vi "ep_Build Waveforms (Multiple Lines).vi"(5 "reset? (F)":bool, 6 "current channels":T1[](array[typedef]) {"physical channels"."channel phase" items=["Phase A (L1)", "Phase B (L2)", "Phase C (L3)", "Phase N (Neutral)"]}, 7 "t0":timestamp, 8 "error in (no error)":errorcluster, 9 "voltage channels":T1[](array[typedef]) {"physical channels"."channel phase" items=["Phase A (L1)", "Phase B (L2)", "Phase C (L3)", "Phase N (Neutral)"]}, 10 "dt":dbl, 11 "AI data":sgl[][](array[numeric]) format="%#.21g") -> (0 "error out":errorcluster, 2 "current waveforms":waveform(sgl)[](array[waveform]), 3 "voltage waveforms":waveform(sgl)[](array[waveform]))   [LabVIEW 2014, in "NI_EP_Power Quality.lvlib"]
uses:
  <vilib>/addons/Electrical Power/PQ/NI_EP_Power Quality.lvlib
  <vilib>/addons/Electrical Power/PQ/Common/Controls/ep_Channels Config.ctl
  <vilib>/addons/Electrical Power/PQ/Common/Controls/ep_Channel Phase.ctl
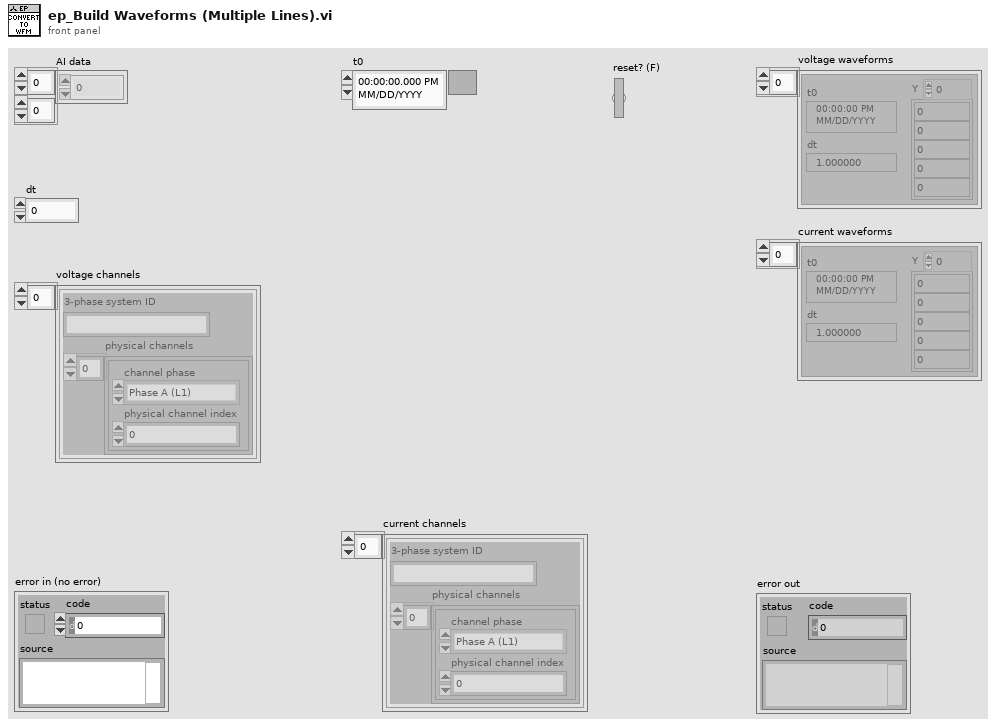
[diagram p1: front panel]
types:
  T1 = typedef "NI_EP_Power Quality.lvlib/ep_Channels Config.ctl" = cluster{"3-phase system ID":string, "physical channels":cluster{"channel phase":T2, "physical channel index":u16}[]}
  T2 = typedef "NI_EP_Power Quality.lvlib/ep_Channel Phase.ctl" = u16
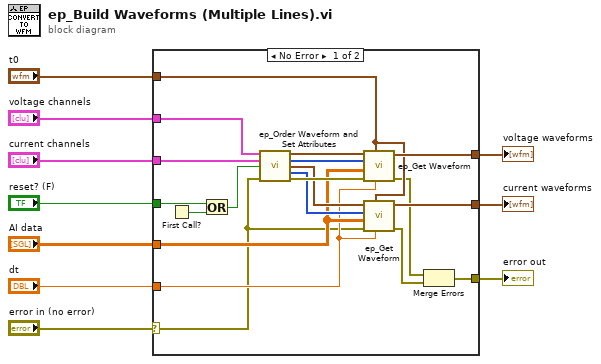
[diagram p0: block diagram]
diagram:
  n1 = case shown="No Error" "error in (no error)" {
    selector: "error in (no error)" -> [w11 w30]
    tunnel: "reset? (F)" -> [w29 _]
    tunnel: "voltage channels" -> [w27 _]
    tunnel: "current channels" -> [w26 _]
    tunnel: [w21 _] -> w9
    tunnel: "AI data" -> [w18 _]
    tunnel: "dt" -> [w17 _]
    tunnel: "t0" -> [w16 _]
    tunnel: [w15 _] -> w5
    tunnel: [w12 w30] -> w4
    frame No Error {
      n2 = First Call?() -> (First Call?: T/F=w28:bool)
      n3 = Or(x=w29, y=w28) -> (x .or. y?=w25:bool)
      n4 = call <vilib>:"ep_Order Waveform and Set Attributes.vi"("voltage channels"=w27, "current channels"=w26, "reset? (F)"=w25, "error in (no error)"=w11) -> ("voltage waveforms"=w24:waveform(sgl)[], "voltage physical channel indexes"=w23:u16[], "current waveforms"=w20:waveform(sgl)[], "current physical channel indexes"=w19:u16[], "error out"=w22:errorcluster)  [unwired: 7 in]
      n5 = call <vilib>:"ep_Get Waveform.vi"("dt"=w17, "t0"=w16, "error in (no error)"=w22, "AI data"=w18, "physical channel indexes"=w23, "waveform in"=w24) -> ("error out"=w14:errorcluster, "waveform out"=w21:waveform(sgl)[])  [unwired: 4 in]
      n6 = call <vilib>:"ep_Get Waveform.vi"("dt"=w17, "t0"=w16, "error in (no error)"=w11, "AI data"=w18, "physical channel indexes"=w19, "waveform in"=w20) -> ("error out"=w13:errorcluster, "waveform out"=w15:waveform(sgl)[])  [unwired: 4 in]
      n7 = Merge Errors(w14, w13) -> (w12:errorcluster)
    }
    frame Error {
    }
  }
  "voltage waveforms" <- w9
  "error out" <- w4
  "current waveforms" <- w5
